vi "Write Local Resource.vi"(8 "error in (no error)":errorcluster, 10 "Local Resource":refnum<visa-resource-name>, 11 "6700C in":refnum<class "6700C.lvclass">) -> (0 "error out":errorcluster, 3 "6700C out":refnum<class "6700C.lvclass">)   [LabVIEW 2019, in "6700C.lvlib" / "6700C.lvclass"]
uses:
  Library/6700C.lvclass
  Library/6700C.lvclass/6700C.ctl
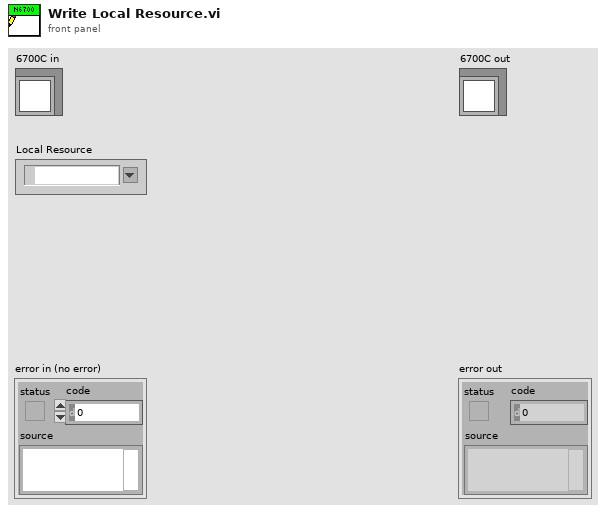
[diagram p1: front panel]
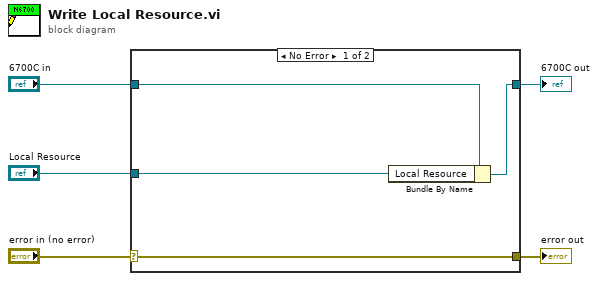
[diagram p0: block diagram]
diagram:
  n1 = case shown="No Error" "error in (no error)" {
    selector: "error in (no error)" -> [w9 w10]
    tunnel: [w9 w10] -> w4
    tunnel: [w7 w11] -> w2
    tunnel: "6700C in" -> [w8 w11]
    tunnel: "Local Resource" -> [w6 _]
    frame No Error {
      n2 = Bundle By Name(cluster=w8, "Local Resource"=w6) -> (w7:refnum<class "6700C.lvclass">)
    }
    frame Error {
    }
  }
  "error out" <- w4
  "6700C out" <- w2
